vi "Read RotPA.lvclass.vi"(8 "error in (no error)":errorcluster, 11 "RotatorPositions.lvclass in":refnum<class "RotatorPositions.lvclass">) -> (0 "error out":errorcluster, 2 "RotPA.lvclass":refnum<class "RotPA.lvclass">, 3 "RotatorPositions.lvclass out":refnum<class "RotatorPositions.lvclass">)   [LabVIEW 2009]
uses:
  RotatorPositions.lvclass
  TCSCommand/TargetConfiguration/Rotator/RotPA/RotPA.lvclass
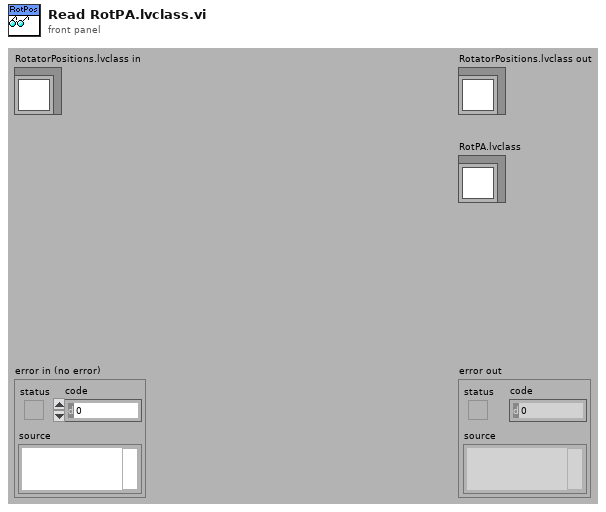
[diagram p1: front panel]
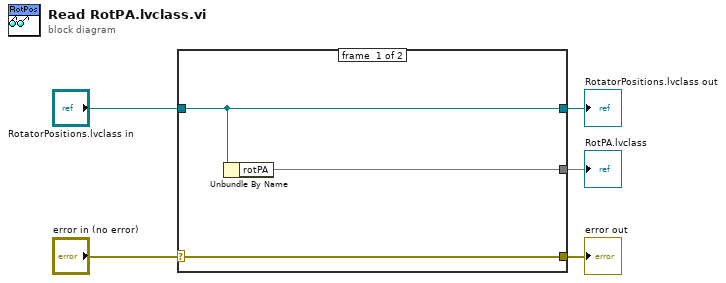
[diagram p0: block diagram]
diagram:
  n1 = case shown="No Error" "error in (no error)" {
    selector: "error in (no error)" -> [w8 w9]
    tunnel: [w8 w9] -> w4
    tunnel: [w7 w10] -> w2
    tunnel: "RotatorPositions.lvclass in" -> [w7 w10]
    tunnel: [w6 _] -> w1
    frame #0 {
      n2 = Unbundle By Name(w7) -> ("rotPA"=w6)
    }
    frame #1 {
    }
  }
  "error out" <- w4
  "RotatorPositions.lvclass out" <- w2
  "RotPA.lvclass" <- w1
